vi "Reset Yaw.vi"(1 "Reset":bool) -> ()   [LabVIEW 2023]
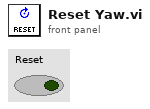
[diagram p1: front panel]
types:
  T1 = typedef "CTRE_PigeonIMU_DeviceRef.ctl" = cluster{"DeviceStatus":errorcluster, "Device Number":u8, "Type":T2, "Device ID":u32, "Handle":u64, "UsageFrame":u32, "Library Path":path}
  T2 = typedef "CTRE_PigeonIMU_ConnectionType.ctl" = u32
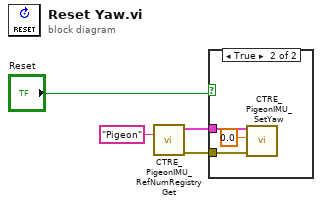
[diagram p0: block diagram]
diagram:
  n1 = call <vilib>:"CTRE_PigeonIMU_RefNumRegistryGet.vi"("refnum name"="Pigeon") -> ("error out"=w2:errorcluster, "PigeonIMUDevRef"=w3:T1)  [unwired: 9 in]
  n2 = case shown="True" "Reset" {
    tunnel: w3 -> [_ w7]
    tunnel: w2 -> [_ w6]
    frame False {
    }
    frame True {
      n3 = call <vilib>:"CTRE_PigeonIMU_SetYaw.vi"("error in (no error)"=w6, "Value"=0.0, "PigeonIMUDevRef"=w7) -> ()  [unwired: 7 in, 2 out]
    }
  }
